vi "RtdeIsNewOutputDataAvailable.vi"(8 "Rtde":refnum<k24>, 11 "error in":errorcluster) -> (0 "Data available":bool, 3 "error out":errorcluster)   [LabVIEW 2022 SP3, in "UnderAutomation.UniversalRobots.lvlib"]
uses:
  UnderAutomation.UniversalRobots.lvlib
  C:/Users/fg/Documents/UniversalRobots.vi/LabVIEW_2023/UnderAutomation.UniversalRobots/lib/UnderAutomation.UniversalRobots.dll
  LabVIEW_2023/UnderAutomation.UniversalRobots/lib/UnderAutomation.UniversalRobots.dll
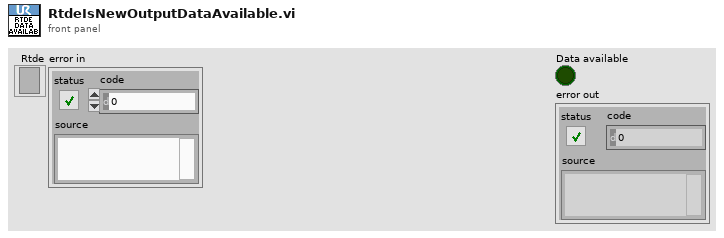
[diagram p1: front panel]
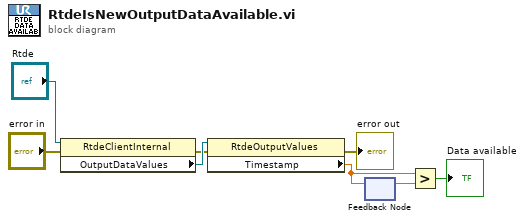
[diagram p0: block diagram]
diagram:
  n1 = property class="RtdeClientInternal"(reference="Rtde", error in="error in") -> (error out=w3:errorcluster, "OutputDataValues"=w7:refnum<k24>)  [unwired: 1 out]
  n2 = property class="RtdeOutputValues"(reference=w7, error in=w3) -> (error out=→"error out":errorcluster, "Timestamp"=w6:dbl)  [unwired: 1 out]
  n3 = feedback #1() -> (w5:dbl)  [unwired: 1 in]
  n4 = feedback-in #1(w6) -> ()
  n5 = Greater?(x=w6, y=w5) -> (0:→"Data available":bool)
